vi "AK Befehl Auswerten_v1.2.vi"(10 "Array":string[](array[string])) -> (2 "String für schreiben":string)   [LabVIEW 2020, in "AK-Schnittstelle.lvlib"]
uses:
  AK-Schnittstelle.lvlib
  Aktionen Stoernummern pruefen.ctl
  Aktionen Zustandsfehlerinformation.ctl
  Funktionstasten/Zustaende.ctl
  Funktionstasten/Funktionstasten.lvlib
  Funktionstasten/Betriebsart.ctl
  Funktionstasten/Funktionstasten-Aktion.ctl
  Aktionen Gespeicherte Werte.ctl
  Seiten/Log Konfig/LogKonfig.lvlib
  Seiten/Log Konfig/Aktionen Trigger.ctl
  Seiten/FT-IR/FT-IR.lvlib
  Seiten/FT-IR/FGV FT-IR Gasliste Aktionen.ctl
  Messdaten/Messdaten.lvlib
  Messdaten/Aktionen FGV Messdaten.ctl
  Seiten/System Einstellungen V2/System Einstellungen V2.lvlib
  Seiten/System Einstellungen V2/Aktioen FGV System Konstanten.ctl
  Seiten/Erweiterte Konfig/FGV PID Aktionen.ctl
  Seiten/Erweiterte Konfig/Erweiterte Konfig.lvlib
  Seiten/Erweiterte Konfig/Dichtheitstest.vi
  Allgemein/allgemeine Sub-VIs.lvlib
  cRIO/PC/Kommunikation mit cRIO.lvlib
  Seiten/FT-IR/FGV FT-IR Diagnose Aktionen.ctl
  Seiten/Erweiterte Konfig/Status Dichtheitstest Aktionen.ctl
  Seiten/FT-IR/FGV FT-IR Aktionen.ctl
  Seiten/Anlagengrenzwerte/Anlagengrenzwerte.lvlib
  Seiten/Anlagengrenzwerte/FGV Anlagengrenzwerte Aktionen.ctl
  Seiten/FT-IR/TOOLweb Interface Library/TOOLweb Interface.lvlib
  Seiten/System Einstellungen V2/Aktioen FGV System.ctl
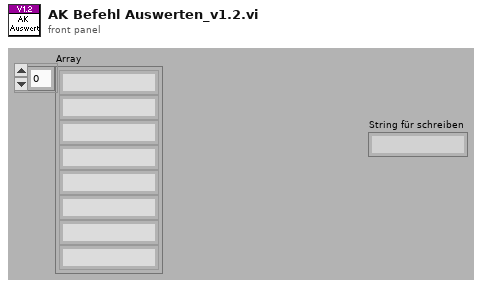
[diagram p1: front panel]
types:
  T1 = typedef "AK-Schnittstelle.lvlib/Aktionen Stoernummern pruefen.ctl" = enum16{"lesen", "prüfen"}
  T2 = typedef "AK-Schnittstelle.lvlib/Aktionen Zustandsfehlerinformation.ctl" = enum16{"OK", "Offline", "Busy", "Syntax Error", "Datenfehler"}
  T3 = typedef "AK-Schnittstelle.lvlib/Aktionen Gespeicherte Werte.ctl" = enum16{"lesen", "laden", "speichern", "Seriell", "TCP", "Diverse", "AKTIV", "AK-Namen"}
  T4 = typedef "System Einstellungen V2.lvlib/Aktioen FGV System Konstanten.ctl" = enum16{"lesen", "laden", "speichern", "Sprache"}
  T5 = typedef "Messdaten.lvlib/Aktionen FGV Messdaten.ctl" = enum16{"lesen", "schreiben", "löschen", "Mittelwerte", "Komponente"}
  T6 = typedef "System Einstellungen V2.lvlib/Aktioen FGV System.ctl" = enum16{"lesen", "laden", "speichern", "Optionen schreiben", "Zeitstempel", "Reset BMP", "Reset SQP", "Wartung", "Werkseinstellung"}
  T7 = typedef "Funktionstasten.lvlib/Funktionstasten-Aktion.ctl" = enum16{"Initialisieren", "Zustand setzen", "Taste gedrückt", "Fehler speichern", "Lesen", "Manuell", "Remote", "Bitparallel", "Samplepoint", "Zeit Prüfen", "reset Umschalten"}
  T8 = typedef "FT-IR.lvlib/FGV FT-IR Gasliste Aktionen.ctl" = enum16{"lesen", "Gasliste FT-IR", "Gasliste ausgelesen", "laden", "speichern", "löschen"}
  T9 = typedef "FT-IR.lvlib/FGV FT-IR Diagnose Aktionen.ctl" = enum16{"Lesen", "Diagnose Schreiben", "Min Schreiben", "Max Schreiben"}
  T10 = typedef "Erweiterte Konfig.lvlib/Status Dichtheitstest Aktionen.ctl" = enum16{"lesen", "Zeitstempel", "Daten", "läuft", "Protokolldaten"}
  T11 = typedef "Erweiterte Konfig.lvlib/FGV PID Aktionen.ctl" = enum16{"Lesen", "Schreiben PID", "Schreiben Sonstige", "Dichtheitstest", "Aktionen Dicht.", "Parameter Sensor"}
  T12 = typedef "FT-IR.lvlib/FGV FT-IR Aktionen.ctl" = enum16{"lesen", "NOG setzen", "NOS setzen", "Initialisieren", "speichern", "ALLES setzen", "FT-IR Spektrum loggen", "Komm Stoppen", "Spektrum LogKonfig"}
  T13 = typedef "Anlagengrenzwerte.lvlib/FGV Anlagengrenzwerte Aktionen.ctl" = enum16{"Lesen", "Grenzwerte schreiben"}
  T14 = typedef "Funktionstasten.lvlib/Zustaende.ctl" = enum16{"Standby", "Pause", "Eco", "Messen", "Kalibrieren", "Spülen Filter", "Spülen Leitung", "Umgebungsluft", "0-Gas", "Cal-Gas", "CG zu PNS", "-------------", "Init 1", "Init 2", "Init 3", "Init 4", "Messen vorbereiten", "Messen durchführen", "Exit"}
  T15 = typedef "Funktionstasten.lvlib/Betriebsart.ctl" = enum16{"Manuell", "Remote", "Bitparallel"}
  T16 = typedef "Funktionstasten.lvlib/Zustaende.ctl" = enum16{"Standby", "Pause", "Eco", "Messen", "Kalibrieren", "Spülen Filter", "Spülen Leitung", "Umgebungsluft", "0-Gas", "Cal-Gas 1", "-------------", "Init 1", "Init 2", "Init 3", "Init 4", "Messen vorbereiten", "Messen durchführen", "Exit"}
  T17 = typedef "LogKonfig.lvlib/Aktionen Trigger.ctl" = enum16{"lesen", "ALLE schreiben", "Trigger prüfen", "Trigger rücksetzen"}
  T18 = typedef "AK-Schnittstelle.lvlib/Diverse gespeicherte Werte.ctl" = cluster{"Kalibriergaseingang":i16, "SamplePoint":i16, "CalGas zu PNS":i16, "Gas-Reihenfolge":i16[], "Zeit 0-Gas":sgl, "Zeit CalGas":sgl, "AK Befehlssatz":T19}
  T19 = typedef "AK-Schnittstelle.lvlib/AK Befehlssatz.ctl" = enum16{"MEXA", "IAG v1.4", "AVL (Puma)", "PEUS"}
  T20 = typedef "System Einstellungen.lvlib/Optionen.ctl" = cluster{"Störmeldep.":bool, "Betriebszustände":bool, "LN2 Befüllung":bool, "Klimaanlage ?":bool, "AK in ppm":bool, "log Cal-Gas":bool, "log 0-Gas":bool, "log CG zu PNS":bool, "Reserve":bool, "Reserve1":bool, "PNS?":bool, "Container":bool, "Mit N2 spülen":bool, "Span Gas Auswahl":T21}
  T21 = typedef "Funktionstasten.lvlib/Spaneingang.ctl" = u16
  T22 = typedef "String - Ausgabefeld.ctl" = string
  T23 = cluster{"AI0: Durchfluss FT-IR":sgl, "AI1: Druck Ausgang":sgl, "AI2: Umgebungsdruck":sgl, "AI3: Druck FT-IR":sgl, "AI4: Druck CalGas":sgl, "AI5: Reserve":sgl, "AI6: Reserve":sgl, "AI7: Reserve":sgl, "Rohwert Durchfluss FT-IR":sgl, "Rohwert Druck Ausgang":sgl, "Rohwert Umgebungsdruck":sgl, "Rohwert Druck FT-IR":sgl, "Rohwert Durchfluss M":sgl, "TC0: Schaltschrank":sgl, "TC1: Filter":sgl, "TC2: Pumpe":sgl, "TC3: HL BMP zu Filter":sgl, "TC4: HL zu FT-IR":sgl, "TC5: HL Extern SP1":sgl, "TC6: HL Extern SP2":sgl, "TC7: Heizung Extern 1":sgl, "TC8: Heizung Extern 2":sgl, "TC9: Reserve":sgl, "TC10: Reserve":sgl, "TC11: Reserve":sgl, "TC12: FT-IR":sgl, "TC13: Reserve":sgl, "TC14: Reserve":sgl, "TC15: Reserve":sgl}
  T24 = typedef "Erweiterte Konfig.lvlib/Sonstige Parameter.ctl" = cluster{"Lüfter langsam":sgl, "Lüfter schnell":sgl, "FT-IR Kühlung Soll":sgl, "FT-IR Kühlung Max":sgl, "Überwachung":T25, "Befüllung aktiv":T26, "Stickstoff Befüllzeit":sgl, "Befüllintervall":sgl, "Kalibrierwert FT-IR":sgl, "Offset Ausgang":sgl, "Offset FT-IR":sgl, "Offset Druck FT-IR":sgl, "Dichtheitstest Zeit":sgl, "Dichtheitstest Abfall":sgl, "Dichtheitstest Umfang":T27, "Offset Umgebung":sgl, "Max Taupunkt":sgl, "Pumpendrehzahl":sgl, "ext. Befüllung":T26, "Ext. Stickstoff Befüllzeit":sgl}
  T25 = typedef "Auswahlfeld.ctl" = u16
  T26 = typedef "LogKonfig.lvlib/Auswahlfeld aktiviert-deaktiviert.ctl" = u16
  T27 = typedef "Erweiterte Konfig.lvlib/Dichtheitstest Umfang.ctl" = u16
  T28 = typedef "Anlagengrenzwerte.lvlib/Anlagen-Grenzwerte Anzeige.ctl" = cluster{"Eingangsdruck FT-IR:":T29, "Durchfluss FT-IR:":T29, "Durchfluss CalGas:":T29, "Druck Ausgang:":T29, "Druck Kalter Block:":T29, "Heizleitungen intern:":T29, "Heizleitung zu FT-IR:":T29, "Heizung Filterblock:":T29, "Heizung Pumpe:":T29, "Heizleitung Extern SP1:":T29, "Heizleitung Extern SP2:":T29, "FT-IR Heizung Messzelle:":T29, "Schaltschranktemperatur:":T29, "Gaskühler:":T29}
  T29 = typedef "Anlagengrenzwerte.lvlib/Anlagen-Parameter Anzeige.ctl" = cluster{"Sollwert":sgl, "Warn-Min":sgl, "Warn-Max":sgl, "Abschalt-Min":sgl, "Abschalt-Max":sgl, "Regler":u16}
  T30 = typedef "LogKonfig.lvlib/Element Triggerereignisse.ctl" = cluster{"Trigger verwenden":T26, "Messwert":u16, "kl./gr.":u16, "Wert":sgl, "Puffergröße":sgl}
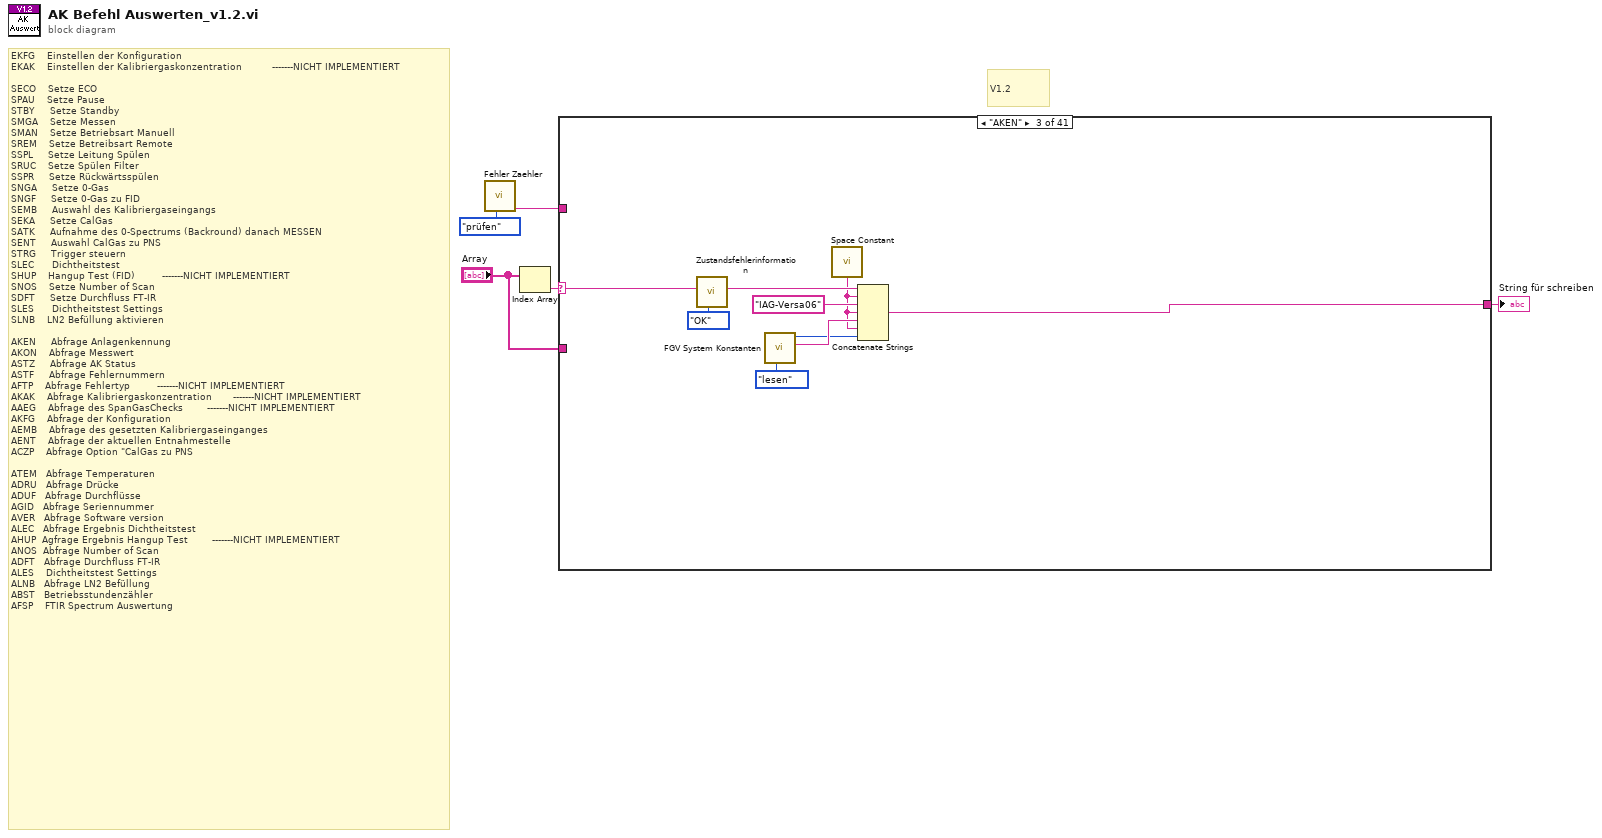
[diagram p0: block diagram]
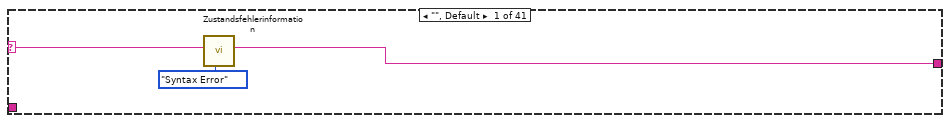
[diagram p2: hidden frame]
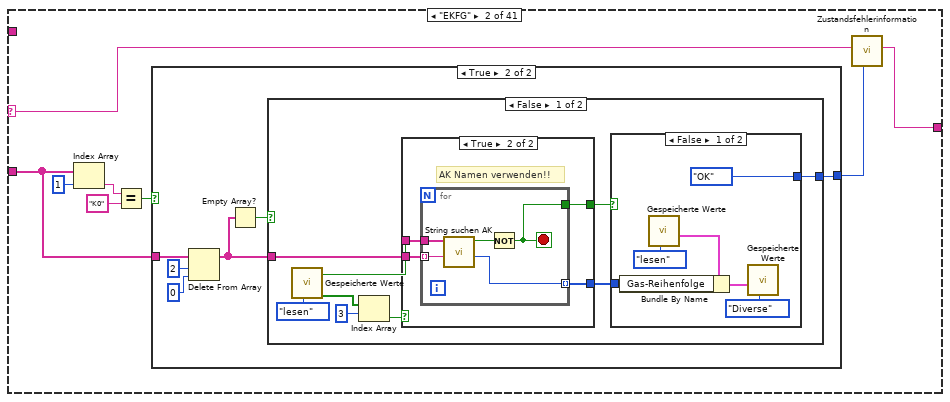
[diagram p3: hidden frame]
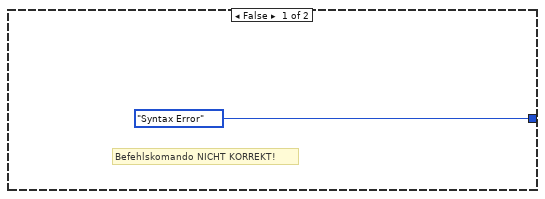
[diagram p4: hidden frame]
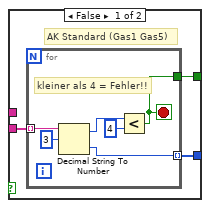
[diagram p5: hidden frame]
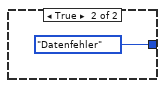
[diagram p6: hidden frame]
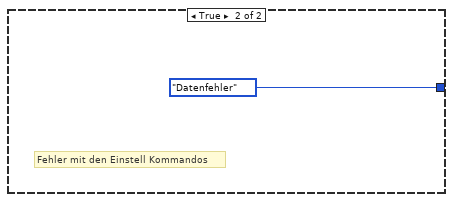
[diagram p7: hidden frame]
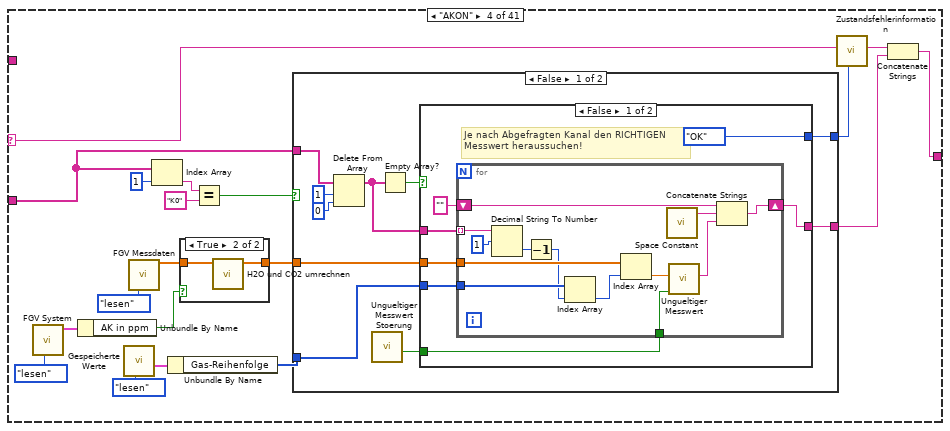
[diagram p8: hidden frame]
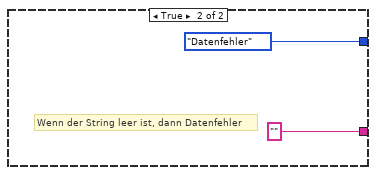
[diagram p10: hidden frame]
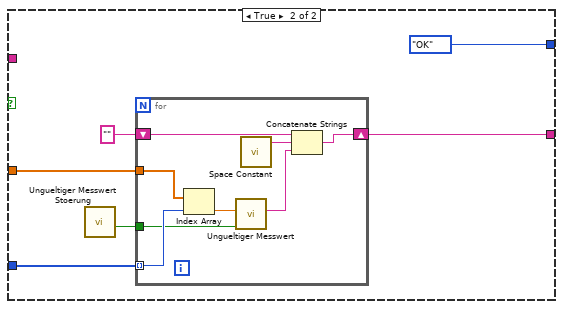
[diagram p11: hidden frame]
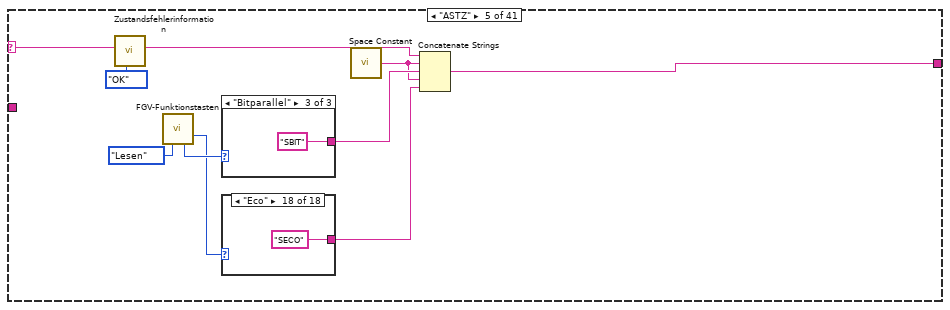
[diagram p12: hidden frame]
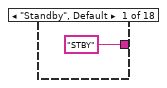
[diagram p13: hidden frame]
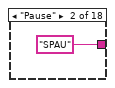
[diagram p14: hidden frame]
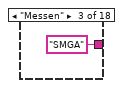
[diagram p15: hidden frame]
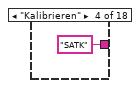
[diagram p16: hidden frame]
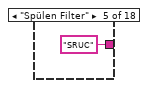
[diagram p17: hidden frame]
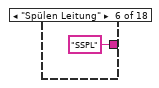
[diagram p18: hidden frame]
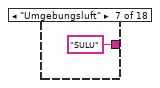
[diagram p19: hidden frame]
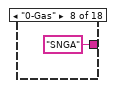
[diagram p20: hidden frame]
diagram:
  # "V1.2"
  # "EKFG    Einstellen der Konfiguration\nEKAK    Einstellen der Kalibriergaskonzentration          -------NICHT IMPLEMENTIERT\n\nSECO    Setze ECO\nSPAU    Setze Pause\nSTBY     Setze Standby\nSMGA    Setze Messen\nSMAN    Setze Betriebsart Manuell\nSREM    Setze Betreibsart Remote\nSSPL     Setze Leitung Spülen\nSRUC    Setze Spülen Filter\nSSPR     Setze Rückwärtsspülen\nSNGA     Setze 0-Gas\nSNGF     Setze 0-Gas zu FID\nSEMB     Auswahl des Kalibriergaseingangs\nSEKA     Setze CalGas\nSATK     Aufnahme des 0-Spectrums (Backround) danach MESSEN\nSENT     Auswahl CalGas zu PNS\nSTRG     Trigger steuern\nSLEC      Dichtheitstest\nSHUP    Hangup Test (FID)         -------NICHT IMPLEMENTIERT\nSNOS    Setze Number of Scan\nSDFT     Setze Durchfluss FT-IR\nSLES      Dichtheitstest Settings\nSLNB    LN2 Befüllung aktivieren\n\nAKEN     Abfrage Anlagenkennung\nAKON    Abfrage Messwert\nASTZ     Abfrage AK Status\nASTF     Abfrage Fehlernummern\nAFTP    Abfrage Fehlertyp         -------NICHT IMPLEMENTIERT\nAKAK    Abfrage Kalibriergaskonzentration       -------NICHT IMPLEMENTIERT\nAAEG    Abfrage des SpanGasChecks        -------NICHT IMPLEMENTIERT\nAKFG    Abfrage der Konfiguration\nAEMB    Abfrage des gesetzten Kalibriergaseinganges\nAENT    Abfrage der aktuellen Entnahmestelle\nACZP    Abfrage Option \"CalGas zu PNS\n\nATEM   Abfrage Temperaturen\nADRU   Abfrage Drücke\nADUF   Abfrage Durchflüsse\nAGID   Abfrage Seriennummer\nAVER   Abfrage Software version\nALEC   Abfrage Ergebnis Dichtheitstest\nAHUP  Agfrage Ergebnis Hangup Test        -------NICHT IMPLEMENTIERT\nANOS  Abfrage Number of Scan\nADFT   Abfrage Durchfluss FT-IR\nALES    Dichtheitstest Settings\nALNB   Abfrage LN2 Befüllung\nABST   Betriebsstundenzähler\nAFSP    FTIR Spectrum Auswertung"
  n1 = call "Fehler Zaehler.vi"("Aktionen"=Aktionen_Stoernummern_pruefen."prüfen") -> ("Fehlerzähler"=w3:string)  [unwired: 7 in, 3 out]
  n2 = Index Array(array="Array") -> (element=w2:string)  [unwired: 1 in]
  n3 = case shown="\"AKEN\"" w2 {
    selector: w2 -> [w7 w15 w65 w85 w143 w163 w176 w223 w232 w241 w257 w280 w294 w301 w308 w323 w344 w355 w364 w374 w388 w396 w399 w402 w405 w415 w425 w429 w439 w443 w445 w458 w463 w484 w503 w507 w529 w568 w592 w643 w674]
    tunnel: [w6 w14 w67 w86 w145 w165 w178 w225 w234 w243 w245 w275 w291 w296 w304 w316 w342 w357 w366 w376 w386 w395 w398 w401 w404 w414 w424 w428 w438 w442 w444 w457 w462 w483 w502 w506 w528 w567 w591 w642 w673] -> w5
    tunnel: w3 -> [_ _ _ _ _ _ _ _ _ _ _ _ _ _ _ _ _ _ _ _ _ _ _ _ _ _ _ _ _ _ _ _ _ _ _ _ _ _ _ _ _]
    tunnel: "Array" -> [_ w16 _ w76 _ _ _ _ _ _ _ _ _ _ _ _ _ _ _ _ _ _ _ _ _ w407 w417 _ w437 _ _ _ w461 _ _ w505 w527 _ w590 w641 w672]
    frame "", Default {
      n4 = call "Zustandsfehlerinformation.vi"("Aktionen"=Aktionen_Zustandsfehlerinformation."Syntax Error", "String"=w7) -> ("String"=w6:string)  [unwired: 9 in]
    }
    frame "EKFG" {
      n5 = Index Array(array=w16, index=1 ("Index")) -> (element=w12:string)
      n6 = Equal?(x=w12, y="K0") -> (x = y?=w10:bool)
      n7 = case shown="True" w10 {
        tunnel: w16 -> [_ w21]
        tunnel: [Aktionen_Zustandsfehlerinformation."Syntax Error" ("Aktionen") w18] -> w9
        frame False {
          # "Befehlskomando NICHT KORREKT!"
        }
        frame True {
          n8 = Delete From Array(array=w21, length=2 ("Länge"), index=0 ("Index")) -> (array with subset deleted=w20:string[])  [unwired: 1 out]
          n9 = Empty Array?(array=w20) -> (empty?=w19:bool)
          n10 = case shown="False" w19 {
            tunnel: w20 -> [w32 _]
            tunnel: [w28 Aktionen_Zustandsfehlerinformation."Datenfehler" ("Aktionen")] -> w18
            frame False {
              n11 = call "Gespeicherte Werte.vi"("Aktionen"=Aktionen_Gespeicherte_Werte."lesen") -> ("AKTIV?"=w25:bool[], "Port changed in"=w29:bool)  [unwired: 5 in, 4 out]
              n12 = Index Array(array=w25, index=3 ("Index")) -> (element=w24:bool)
              n13 = case shown="True" w24 {
                tunnel: w32 -> [w33 w45]
                tunnel: [w34 w44] -> w31
                tunnel: w29 -> [_ w43]
                tunnel: [w35 w42] -> w27
                frame False {
                  # "AK Standard (Gas1 Gas5)"
                  n14 = for {
                    tunnel: w33 -> [w40] mode=indexing
                    tunnel: [w39] -> w34 mode=indexing
                    tunnel: [w36] -> w35
                    stop <- w36 stop-if-true
                    # "kleiner als 4 = Fehler!!"
                    n15 = Decimal String To Number(string=w40, offset=3 ("Offset")) -> (offset past number=w37:i32, number=w39:i32)  [unwired: 1 in]
                    n16 = Less?(x=w37, y=4) -> (x < y?=w36:bool)
                  }
                }
                frame True {
                  # "AK Namen verwenden!!"
                  n17 = for {
                    tunnel: w45 -> [w48] mode=indexing
                    tunnel: [w47] -> w44 mode=indexing
                    tunnel: w43 -> [w49]
                    tunnel: [w50] -> w42
                    stop <- w50 stop-if-true
                    n18 = call "String suchen AK.vi"("gesucht"=w48, "Namen"=w49) -> ("Index"=w47:i32, "Gefunden?"=w46:bool)  [unwired: 8 in]
                    n19 = Not(x=w46) -> (.not. x?=w50:bool)
                  }
                }
              }
              n20 = case shown="False" w27 {
                tunnel: w31 -> [w55 _]
                tunnel: [Aktionen_Zustandsfehlerinformation."OK" ("Aktionen") Aktionen_Zustandsfehlerinformation."Datenfehler" ("Aktionen")] -> w28
                frame False {
                  n21 = call "Gespeicherte Werte.vi"("Aktionen"=Aktionen_Gespeicherte_Werte."lesen") -> ("Diverse Werte"=w53:T18)  [unwired: 6 in, 4 out]
                  n22 = Bundle By Name(cluster=w53, "Gas-Reihenfolge"=w55) -> (w52:T18)
                  n23 = call "Gespeicherte Werte.vi"("Aktionen"=Aktionen_Gespeicherte_Werte."Diverse", "Diverse Werte"=w52) -> ()  [unwired: 5 in, 5 out]
                }
                frame True {
                }
              }
            }
            frame True {
              # "Fehler mit den Einstell Kommandos"
            }
          }
        }
      }
      n24 = call "Zustandsfehlerinformation.vi"("Aktionen"=w9, "String"=w15) -> ("String"=w14:string)  [unwired: 9 in]
    }
    frame "AKEN" {
      n25 = call "Zustandsfehlerinformation.vi"("Aktionen"=Aktionen_Zustandsfehlerinformation."OK", "String"=w65) -> ("String"=w64:string)  [unwired: 9 in]
      n26 = call "FGV System Konstanten.vi"("Aktionen"=Aktioen_FGV_System_Konstanten."lesen") -> ("LanguageList"=w62:string, "Sprachindex"=w61:u16)  [unwired: 6 in, 3 out]
      n27 = call <vilib>:"Space Constant.vi"() -> ("String"=w59:string)
      n28 = Concatenate Strings(w64, w59, "IAG-Versa06" ("String"), w59, w62, w59, w61) -> (w67:string)
    }
    frame "AKON" {
      n29 = call "FGV System.vi"("Aktionen"=Aktioen_FGV_System."lesen") -> ("Optionen"=w70:T20)  [unwired: 8 in, 2 out]
      n30 = Unbundle By Name(w70) -> ("AK in ppm"=w73:bool)
      n31 = call "Gespeicherte Werte.vi"("Aktionen"=Aktionen_Gespeicherte_Werte."lesen") -> ("Diverse Werte"=w74:T18)  [unwired: 6 in, 4 out]
      n32 = call "FGV Messdaten.vi"("Aktionen"=Aktionen_FGV_Messdaten."lesen") -> ("Aktuelle Messwerte"=w72:sgl[])  [unwired: 6 in, 8 out]
      n33 = Index Array(array=w76, index=1 ("Index")) -> (element=w79:string)
      n34 = Unbundle By Name(w74) -> ("Gas-Reihenfolge"=w82:i16[])
      n35 = case shown="True" w73 {
        tunnel: w72 -> [w87 w89]
        tunnel: [w87 w88] -> w69
        frame False {
        }
        frame True {
          n36 = call "H2O und CO2 umrechnen.vi"("Aktuelle Messwerte"=w89) -> ("Aktuelle Messwerte"=w88:sgl[])  [unwired: 10 in]
        }
      }
      n37 = Equal?(x=w79, y="K0") -> (x = y?=w77:bool)
      n38 = case shown="False" w77 {
        tunnel: w82 -> [w93 w127]
        tunnel: [w91 w125] -> w81
        tunnel: w69 -> [w92 w124]
        tunnel: w76 -> [w97 _]
        tunnel: [w95 Aktionen_Zustandsfehlerinformation."OK" ("Aktionen")] -> w75
        frame False {
          n39 = Delete From Array(array=w97, length=1 ("Länge"), index=0 ("Index")) -> (array with subset deleted=w94:string[])  [unwired: 1 out]
          n40 = call "Ungueltiger Messwert Stoerung.vi"() -> ("Störung Messgerät"=w90:bool)  [unwired: 11 in]
          n41 = Empty Array?(array=w94) -> (empty?=w96:bool)
          n42 = case shown="False" w96 {
            tunnel: [Aktionen_Zustandsfehlerinformation."OK" ("Aktionen") Aktionen_Zustandsfehlerinformation."Datenfehler" ("Aktionen")] -> w95
            tunnel: w94 -> [w105 _]
            tunnel: w93 -> [w104 _]
            tunnel: w92 -> [w103 _]
            tunnel: [w102 ""] -> w91
            tunnel: w90 -> [w100 _]
            frame False {
              # "Je nach Abgefragten Kanal den RICHTIGEN\nMesswert heraussuchen!"
              n43 = for {
                tunnel: w105 -> [w119] mode=indexing
                tunnel: w104 -> [w117]
                tunnel: w103 -> [w116]
                shift-right: [w115] -> w102
                shift-left: "" -> [w114]
                tunnel: w100 -> [w108]
                n44 = Decimal String To Number(string=w119, offset=1 ("Offset (0)")) -> (number=w113:i32)  [unwired: 1 in, 1 out]
                n45 = Decrement(x=w113) -> (x-1=w112:i32)
                n46 = Index Array(array=w117, index=w112) -> (element=w110:i16)
                n47 = Index Array(array=w116, index=w110) -> (element=w109:sgl)
                n48 = call <vilib>:"Space Constant.vi"() -> ("String"=w111:string)
                n49 = call "Ungueltiger Messwert.vi"("Stöung Messgerät"=w108, "Messwert"=w109) -> ("Messwert String"=w107:string)  [unwired: 9 in]
                n50 = Concatenate Strings(w114, w111, w107) -> (w115:string)
              }
            }
            frame True {
              # "Wenn der String leer ist, dann Datenfehler"
            }
          }
        }
        frame True {
          n51 = call "Ungueltiger Messwert Stoerung.vi"() -> ("Störung Messgerät"=w122:bool)  [unwired: 11 in]
          n52 = for {
            tunnel: w127 -> [w131] mode=indexing
            shift-right: [w135] -> w125
            shift-left: "" -> [w134]
            tunnel: w124 -> [w133]
            tunnel: w122 -> [w129]
            n53 = Index Array(array=w133, index=w131) -> (element=w130:sgl)
            n54 = call "Ungueltiger Messwert.vi"("Stöung Messgerät"=w129, "Messwert"=w130) -> ("Messwert String"=w128:string)  [unwired: 9 in]
            n55 = call <vilib>:"Space Constant.vi"() -> ("String"=w132:string)
            n56 = Concatenate Strings(w134, w132, w128) -> (w135:string)
          }
        }
      }
      n57 = call "Zustandsfehlerinformation.vi"("Aktionen"=w75, "String"=w85) -> ("String"=w84:string)  [unwired: 9 in]
      n58 = Concatenate Strings(w84, w81) -> (w86:string)
    }
    frame "ASTZ" {
      n59 = call "Zustandsfehlerinformation.vi"("Aktionen"=Aktionen_Zustandsfehlerinformation."OK", "String"=w143) -> ("String"=w142:string)  [unwired: 9 in]
      n60 = call "FGV-Funktionstasten.vi"("Aktion"=Funktionstasten-Aktion."Lesen") -> ("ausgewählte Funktion"=w138:T14, "Betriebsart"=w140:T15)  [unwired: 7 in, 6 out]
      n61 = case shown="\"Bitparallel\"" w140 {
        tunnel: ["SMAN" ("String") "SREM" ("String") "SBIT" ("String")] -> w139
        frame "Manuell", Default {
        }
        frame "Remote" {
        }
        frame "Bitparallel" {
        }
      }
      n62 = case shown="\"Eco\"" w138 {
        tunnel: ["STBY" ("String") "SPAU" ("String") "SMGA" ("String") "SATK" ("String") "SRUC" ("String") "SSPL" ("String") "SULU" ("String") "SNGA" ("String") "SEKA1" ("String") _ _ _ _ _ _ _ _ "SECO" ("String")] -> w136
        frame "Standby", Default {
        }
        frame "Pause" {
        }
        frame "Messen" {
        }
        frame "Kalibrieren" {
        }
        frame "Spülen Filter" {
        }
        frame "Spülen Leitung" {
        }
        frame "Umgebungsluft" {
        }
        frame "0-Gas" {
        }
        frame "Cal-Gas" {
        }
        frame "Init 1" {
        }
        frame "Init 2" {
        }
        frame "-------------" {
        }
        frame "Init 3" {
        }
        frame "Init 4" {
        }
        frame "Messen vorbereiten" {
        }
        frame "Messen durchführen" {
        }
        frame "Exit" {
        }
        frame "Eco" {
        }
      }
      n63 = call <vilib>:"Space Constant.vi"() -> ("String"=w137:string)
      n64 = Concatenate Strings(w142, w137, w139, w137, w136) -> (w145:string)
    }
    frame "ASTF" {
      n65 = call "Zustandsfehlerinformation.vi"("Aktionen"=Aktionen_Zustandsfehlerinformation."OK", "String"=w163) -> ("String"=w162:string)  [unwired: 9 in]
      n66 = call "Fehler Zaehler.vi"("Aktionen"=Aktionen_Stoernummern_pruefen."lesen") -> ("Fehler Nummern"=w160:string)  [unwired: 7 in, 3 out]
      n67 = call <vilib>:"Space Constant.vi"() -> ("String"=w159:string)
      n68 = Concatenate Strings(w162, w159, w160) -> (w165:string)
    }
    frame "AKFG" {
      n69 = call "Gespeicherte Werte.vi"("Aktionen"=Aktionen_Gespeicherte_Werte."lesen") -> ("Diverse Werte"=w172:T18, "Port changed in"=w170:bool)  [unwired: 5 in, 4 out]
      n70 = Unbundle By Name(w172) -> ("Gas-Reihenfolge"=w174:i16[])
      n71 = disable-structure shown="Deaktiviert" {
        disable-tunnel: [w214 _] -> _
        frame Disabled {
          n72 = call "FGV Gasliste.vi"("Aktionen"=FGV_FT-IR_Gasliste_Aktionen."lesen") -> ("Aktuelle Gasliste gesamt"=w214:T22[])  [unwired: 8 in, 2 out]
        }
        frame Enabled {
        }
      }
      n73 = call "Gespeicherte Werte.vi"("Aktionen"=Aktionen_Gespeicherte_Werte."lesen") -> ("AKTIV?"=w169:bool[])  [unwired: 6 in, 4 out]
      n74 = Index Array(array=w169, index=3 ("Index")) -> (element=w166:bool)
      n75 = case shown="True" w166 {
        tunnel: w174 -> [w188 w205]
        tunnel: [w187 w204] -> w171
        tunnel: w170 -> [w186 _]
        frame True {
          n76 = for {
            tunnel: w188 -> [w194] mode=indexing
            shift-right: [w197] -> w187
            shift-left: "" -> [w196]
            tunnel: w186 -> [w195]
            n77 = Index Array(array=w195, index=w194) -> (element=w192)
            n78 = for {
              N: 15 -> [_]
              shift-right: [w202] -> w191
              shift-left: w192 -> [w203]
              stop <- w200 stop-if-true
              n79 = call <vilib>:"Space Constant.vi"() -> ("String"=w199:string)
              n80 = Search and Replace String(input string=w203, search string=w199, replace string="_") -> (result string=w202:string, number of replacements=w201:i32)  [unwired: 5 in, 2 out]
              n81 = Less Or Equal To 0?(x=w201) -> (x <= 0?=w200:bool)
            }
            n82 = call <vilib>:"Space Constant.vi"() -> ("String"=w190:string)
            n83 = Concatenate Strings(w196, w190, w191) -> (w197:string)
          }
        }
        frame False {
          n84 = for {
            tunnel: w205 -> [w210] mode=indexing
            shift-right: [w213] -> w204
            shift-left: "" -> [w212]
            n85 = Number To Decimal String(number=w210) -> (decimal integer string=w208:string)  [unwired: 1 in]
            n86 = Concatenate Strings("Gas" ("String"), w208) -> (w207:string)
            n87 = call <vilib>:"Space Constant.vi"() -> ("String"=w211:string)
            n88 = Concatenate Strings(w212, w211, w207) -> (w213:string)
          }
        }
      }
      n89 = call "Zustandsfehlerinformation.vi"("Aktionen"=Aktionen_Zustandsfehlerinformation."OK", "String"=w176) -> ("String"=w175:string)  [unwired: 9 in]
      n90 = disable-structure shown="Deaktiviert" {
        disable-tunnel: [w185 _] -> _
        disable-tunnel: _ -> [w184 _]
        disable-tunnel: _ -> [w183 _]
        disable-tunnel: _ -> [w181 _]
        frame Disabled {
          n91 = Number To Decimal String(number=w181) -> (decimal integer string=w179:string)  [unwired: 1 in]
          n92 = call <vilib>:"Space Constant.vi"() -> ("String"=w182:string)
          n93 = Concatenate Strings(w184, w182, w183, w182, "K" ("String"), w179) -> (w185:string)
        }
        frame Enabled {
        }
      }
      n94 = Concatenate Strings(w175, w171) -> (w178:string)
    }
    frame "AEMB" {
      n95 = call "Zustandsfehlerinformation.vi"("Aktionen"=Aktionen_Zustandsfehlerinformation."OK", "String"=w223) -> ("String"=w222:string)  [unwired: 9 in]
      n96 = call "Gespeicherte Werte.vi"("Aktionen"=Aktionen_Gespeicherte_Werte."lesen") -> ("Diverse Werte"=w216:T18)  [unwired: 6 in, 4 out]
      n97 = Unbundle By Name(w216) -> ("Kalibriergaseingang"=w220:i16)
      n98 = call <vilib>:"Space Constant.vi"() -> ("String"=w217:string)
      n99 = Number To Decimal String(number=w220) -> (decimal integer string=w218:string)  [unwired: 1 in]
      n100 = Concatenate Strings(w222, w217, "M" ("String"), w218) -> (w225:string)
    }
    frame "AENT" {
      n101 = call "Zustandsfehlerinformation.vi"("Aktionen"=Aktionen_Zustandsfehlerinformation."OK", "String"=w232) -> ("String"=w231:string)  [unwired: 9 in]
      n102 = call "FGV-Funktionstasten.vi"("Aktion"=Funktionstasten-Aktion."Lesen") -> ("Samplepoint"=w226:u16)  [unwired: 7 in, 7 out]
      n103 = call <vilib>:"Space Constant.vi"() -> ("String"=w228:string)
      n104 = Number To Decimal String(number=w226) -> (decimal integer string=w229:string)  [unwired: 1 in]
      n105 = Concatenate Strings(w231, w228, "M" ("String"), w229) -> (w234:string)
    }
    frame "ACZP" {
      n106 = call "Zustandsfehlerinformation.vi"("Aktionen"=Aktionen_Zustandsfehlerinformation."OK", "String"=w241) -> ("String"=w240:string)  [unwired: 9 in]
      n107 = call "Gespeicherte Werte.vi"("Aktionen"=Aktionen_Gespeicherte_Werte."lesen") -> ("Diverse Werte"=w235:T18)  [unwired: 6 in, 4 out]
      n108 = Unbundle By Name(w235) -> ("CalGas zu PNS"=w238:i16)
      n109 = call <vilib>:"Space Constant.vi"() -> ("String"=w236:string)
      n110 = Number To Decimal String(number=w238) -> (decimal integer string=w237:string)  [unwired: 1 in]
      n111 = Concatenate Strings(w240, w236, w237) -> (w243:string)
    }
    frame "ATEM" {
      n112 = call "Zustandsfehlerinformation.vi"("Aktionen"=Aktionen_Zustandsfehlerinformation."OK", "String"=w257) -> ("String"=w244:string)  [unwired: 9 in]
      n113 = call "FGV cRIO-Daten.vi"("Aktion"=enum16{"lesen", "schreiben"}."lesen") -> ("Analog Input"=w255:T23)  [unwired: 6 in, 8 out]
      n114 = Unbundle By Name(w255) -> ("Rohwert Durchfluss M"=w252:sgl, "TC0: Schaltschrank"=w251:sgl, "TC1: Filter"=w250:sgl, "TC2: Pumpe"=w249:sgl, "TC3: HL BMP zu Filter"=w248:sgl, "TC4: HL zu FT-IR"=w247:sgl)
      n115 = call "FGV FT-IR Diagnosewerte.vi"("Aktionen"=FGV_FT-IR_Diagnose_Aktionen."Lesen") -> ("Temperatur"=w253:dbl)  [unwired: 5 in, 5 out]
      n116 = Build Array(w253, w252, w251, w250, w249, w248, w247) -> (w246:dbl[])
      n117 = for {
        tunnel: w246 -> [w264] mode=indexing
        shift-right: [w259] -> w245
        shift-left: w244 -> [w262]
        n118 = Number To Fractional String(number=w264, precision (6)=i16 1 ("Genauigkeit (6)")) -> (F-format string=w260:string)  [unwired: 2 in]
        n119 = call <vilib>:"Space Constant.vi"() -> ("String"=w261:string)
        n120 = Concatenate Strings(w262, w261, w260) -> (w259:string)
      }
    }
    frame "ADRU" {
      n121 = call "Zustandsfehlerinformation.vi"("Aktionen"=Aktionen_Zustandsfehlerinformation."OK", "String"=w280) -> ("String"=w274:string)  [unwired: 9 in]
      n122 = call "FGV cRIO-Daten.vi"("Aktion"=enum16{"lesen", "schreiben"}."lesen") -> ("Analog Input"=w278:T23)  [unwired: 6 in, 8 out]
      n123 = Unbundle By Name(w278) -> ("AI1: Druck Ausgang"=w270:sgl, "AI3: Druck FT-IR"=w268:sgl)
      n124 = call "FGV FT-IR Diagnosewerte.vi"("Aktionen"=FGV_FT-IR_Diagnose_Aktionen."Lesen") -> ("Druck"=w272:dbl)  [unwired: 5 in, 5 out]
      n125 = Number To Fractional String(number=w272, precision (6)=i16 3 ("Genauigkeit (6)")) -> (F-format string=w267:string)  [unwired: 2 in]
      n126 = Number To Fractional String(number=w270, precision (6)=i16 0 ("Genauigkeit (6)")) -> (F-format string=w265:string)  [unwired: 2 in]
      n127 = Number To Fractional String(number=w268, precision (6)=i16 1 ("Genauigkeit (6)")) -> (F-format string=w266:string)  [unwired: 2 in]
      n128 = Build Array(w267, w265, w266) -> (w276:string[])
      n129 = for {
        tunnel: w276 -> [w282] mode=indexing
        shift-right: [w283] -> w275
        shift-left: w274 -> [w285]
        n130 = call <vilib>:"Space Constant.vi"() -> ("String"=w284:string)
        n131 = Concatenate Strings(w285, w284, w282) -> (w283:string)
      }
    }
    frame "ADUF" {
      n132 = call "Zustandsfehlerinformation.vi"("Aktionen"=Aktionen_Zustandsfehlerinformation."OK", "String"=w294) -> ("String"=w290:string)  [unwired: 9 in]
      n133 = call "FGV cRIO-Daten.vi"("Aktion"=enum16{"lesen", "schreiben"}."lesen") -> ("Analog Input"=w293:T23)  [unwired: 6 in, 8 out]
      n134 = Unbundle By Name(w293) -> ("AI0: Durchfluss FT-IR"=w289:sgl)
      n135 = Number To Fractional String(number=w289, precision (6)=i16 1 ("Genauigkeit (6)")) -> (F-format string=w286:string)  [unwired: 2 in]
      n136 = call <vilib>:"Space Constant.vi"() -> ("String"=w287:string)
      n137 = Concatenate Strings(w290, w287, w286) -> (w291:string)
    }
    frame "AGID" {
      n138 = call "Zustandsfehlerinformation.vi"("Aktionen"=Aktionen_Zustandsfehlerinformation."OK", "String"=w301) -> ("String"=w298:string)  [unwired: 9 in]
      n139 = call "FGV System Konstanten.vi"("Aktionen"=Aktioen_FGV_System_Konstanten."lesen") -> ("LanguageList"=w297:string)  [unwired: 6 in, 4 out]
      n140 = call <vilib>:"Space Constant.vi"() -> ("String"=w300:string)
      n141 = Concatenate Strings(w298, w300, w297) -> (w296:string)
    }
    frame "AVER" {
      n142 = call "Zustandsfehlerinformation.vi"("Aktionen"=Aktionen_Zustandsfehlerinformation."OK", "String"=w308) -> ("String"=w305:string)  [unwired: 9 in]
      n143 = call "FGV System Konstanten.vi"("Aktionen"=Aktioen_FGV_System_Konstanten."lesen") -> ("Sprachindex"=w303:u16)  [unwired: 6 in, 4 out]
      n144 = call <vilib>:"Space Constant.vi"() -> ("String"=w307:string)
      n145 = Concatenate Strings(w305, w307, w303) -> (w304:string)
    }
    frame "ALEC" {
      n146 = call "Zustandsfehlerinformation.vi"("Aktionen"=Aktionen_Zustandsfehlerinformation."OK", "String"=w323) -> ("String"=w322:string)  [unwired: 9 in]
      n147 = call "Status Dichtheitstest.vi"("Aktionen"=Status_Dichtheitstest_Aktionen."lesen") -> ("Fehler"=w311:bool, "läuft?"=w315:bool, "Anstieg"=w320:sgl)  [unwired: 6 in, 2 out]
      n148 = Or(x=w315, y=w311) -> (x .or. y?=w314:bool)
      n149 = Number To Decimal String(number=w320) -> (decimal integer string=w319:string)  [unwired: 1 in]
      n150 = call <vilib>:"Space Constant.vi"() -> ("String"=w318:string)
      n151 = Concatenate Strings(w322, w318, w319) -> (w317:string)
      n152 = Select(t="error", s=w311, f="busy") -> (s? t:f=w310:string)
      n153 = case shown="True" w314 {
        tunnel: w317 -> [w325 w328]
        tunnel: [w325 w326] -> w316
        tunnel: w310 -> [_ w327]
        frame False {
        }
        frame True {
          n154 = call <vilib>:"Space Constant.vi"() -> ("String"=w329:string)
          n155 = Concatenate Strings(w328, w329, w327) -> (w326:string)
        }
      }
    }
    frame "ALES" {
      n156 = call "FGV Erweiterte Konfig.vi"("Aktion"=FGV_PID_Aktionen."Lesen") -> ("Sonstige"=w336:T24)  [unwired: 5 in, 5 out]
      n157 = call "Zustandsfehlerinformation.vi"("Aktionen"=Aktionen_Zustandsfehlerinformation."OK", "String"=w344) -> ("String"=w341:string)  [unwired: 9 in]
      n158 = Unbundle By Name(w336) -> ("Dichtheitstest Zeit"=w333:sgl, "Dichtheitstest Abfall"=w332:sgl, "Dichtheitstest Umfang"=w331:T27)
      n159 = Number To Fractional String(number=w333, precision (6)=i16 0 ("Genauigkeit (6)")) -> (F-format string=w330:string)  [unwired: 2 in]
      n160 = Number To Fractional String(number=w332, precision (6)=i16 0 ("Genauigkeit (6)")) -> (F-format string=w337:string)  [unwired: 2 in]
      n161 = Number To Fractional String(number=w331, precision (6)=i16 0 ("Genauigkeit (6)")) -> (F-format string=w338:string)  [unwired: 2 in]
      n162 = Build Array(w330, w337, w338) -> (w343:string[])
      n163 = for {
        tunnel: w343 -> [w346] mode=indexing
        shift-right: [w347] -> w342
        shift-left: w341 -> [w349]
        n164 = call <vilib>:"Space Constant.vi"() -> ("String"=w348:string)
        n165 = Concatenate Strings(w349, w348, w346) -> (w347:string)
      }
    }
    frame "ANOS" {
      n166 = call "Zustandsfehlerinformation.vi"("Aktionen"=Aktionen_Zustandsfehlerinformation."OK", "String"=w355) -> ("String"=w354:string)  [unwired: 9 in]
      n167 = call "FGV FT-IR Parameter.vi"("Aktion"=FGV_FT-IR_Aktionen."lesen") -> ("NoOfScan"=w350:u32)  [unwired: 11 in, 7 out]
      n168 = call <vilib>:"Space Constant.vi"() -> ("String"=w353:string)
      n169 = Number To Decimal String(number=w350) -> (decimal integer string=w352:string)  [unwired: 1 in]
      n170 = Concatenate Strings(w354, w353, w352) -> (w357:string)
    }
    frame "ALNB" {
      n171 = call "Zustandsfehlerinformation.vi"("Aktionen"=Aktionen_Zustandsfehlerinformation."OK", "String"=w364) -> ("String"=w363:string)  [unwired: 9 in]
      n172 = call "FGV Erweiterte Konfig.vi"("Aktion"=FGV_PID_Aktionen."Lesen") -> ("Sonstige"=w360:T24)  [unwired: 5 in, 5 out]
      n173 = Unbundle By Name(w360) -> ("Befüllung aktiv"=w358:T26)
      n174 = call <vilib>:"Space Constant.vi"() -> ("String"=w362:string)
      n175 = Number To Decimal String(number=w358) -> (decimal integer string=w361:string)  [unwired: 1 in]
      n176 = Concatenate Strings(w363, w362, w361) -> (w366:string)
    }
    frame "ADFT" {
      n177 = call "FGV Anlagengrenzwerte.vi"("Aktion"=FGV_Anlagengrenzwerte_Aktionen."Lesen") -> ("Anlagen-Grenzwerte Anzeige"=w370:T28)  [unwired: 1 in, 9 out]
      n178 = call "Zustandsfehlerinformation.vi"("Aktionen"=Aktionen_Zustandsfehlerinformation."OK", "String"=w374) -> ("String"=w373:string)  [unwired: 9 in]
      n179 = Unbundle By Name(w370) -> ("Durchfluss FT-IR:.Sollwert"=w369:sgl)
      n180 = call <vilib>:"Space Constant.vi"() -> ("String"=w372:string)
      n181 = Number To Fractional String(number=w369, precision (6)=i16 1 ("Genauigkeit (6)")) -> (F-format string=w367:string)  [unwired: 2 in]
      n182 = Concatenate Strings(w373, w372, w367) -> (w376:string)
    }
    frame "ABST" {
      n183 = call "Zustandsfehlerinformation.vi"("Aktionen"=Aktionen_Zustandsfehlerinformation."OK", "String"=w388) -> ("String"=w385:string)  [unwired: 9 in]
      n184 = call "FGV cRIO-Daten.vi"("Aktion"=enum16{"lesen", "schreiben"}."lesen") -> ("PID Stellwerte"=w377:i16[])  [unwired: 6 in, 8 out]
      n185 = Index Array(array=w377) -> (element #1=w378:i16, element #2=w379:i16)  [unwired: 2 in]
      n186 = Number To Fractional String(number=w378, precision (6)=i16 1 ("Genauigkeit (6)")) -> (F-format string=w382:string)  [unwired: 2 in]
      n187 = Number To Fractional String(number=w379, precision (6)=i16 1 ("Genauigkeit (6)")) -> (F-format string=w381:string)  [unwired: 2 in]
      n188 = Build Array(w382, w381) -> (w387:string[])
      n189 = for {
        tunnel: w387 -> [w390] mode=indexing
        shift-right: [w391] -> w386
        shift-left: w385 -> [w393]
        n190 = call <vilib>:"Space Constant.vi"() -> ("String"=w392:string)
        n191 = Concatenate Strings(w393, w392, w390) -> (w391:string)
      }
    }
    frame "SECO" {
      n192 = call "Setze Zustand.vi"("AK Befehl"=w396, "Zustand"=Zustaende."Pause") -> ("Antwort String"=w395:string)  [unwired: 8 in, 1 out]
    }
    frame "SPAU" {
      n193 = call "Setze Zustand.vi"("AK Befehl"=w399, "Zustand"=Zustaende."Pause") -> ("Antwort String"=w398:string)  [unwired: 8 in, 1 out]
    }
    frame "STBY" {
      n194 = call "Setze Zustand.vi"("AK Befehl"=w402, "Zustand"=Zustaende."Standby") -> ("Antwort String"=w401:string)  [unwired: 8 in, 1 out]
    }
    frame "SMGA" {
      n195 = call "Setze Zustand.vi"("AK Befehl"=w405, "Zustand"=Zustaende."Messen") -> ("Antwort String"=w404:string)  [unwired: 8 in, 1 out]
    }
    frame "SSPL" {
      n196 = Index Array(array=w407, index=2 ("Index")) -> (element=w411:string)
      n197 = Decimal String To Number(string=w411) -> (number=w410:i32)  [unwired: 2 in, 1 out]
      n198 = Divide(x=w410, y=10) -> (x/y=w408:dbl)
      n199 = To Single Precision Float(number=w408) -> (single precision float=w406:sgl)
      n200 = call "Setze Zustand.vi"("Zeit"=w406, "AK Befehl"=w415, "Zustand"=Zustaende."Spülen Leitung") -> ("Antwort String"=w414:string)  [unwired: 7 in, 1 out]
    }
    frame "SRUC" {
      n201 = Index Array(array=w417, index=2 ("Index")) -> (element=w421:string)
      n202 = Decimal String To Number(string=w421) -> (number=w420:i32)  [unwired: 2 in, 1 out]
      n203 = Divide(x=w420, y=10) -> (x/y=w418:dbl)
      n204 = To Single Precision Float(number=w418) -> (single precision float=w416:sgl)
      n205 = call "Setze Zustand.vi"("Zeit"=w416, "AK Befehl"=w425, "Zustand"=Zustaende."Spülen Filter") -> ("Antwort String"=w424:string)  [unwired: 7 in, 1 out]
    }
    frame "SSPR" {
      n206 = call "Setze Zustand.vi"("Befehl nicht vorhanden!"=TRUE, "AK Befehl"=w429, "Zustand"=Zustaende."Standby") -> ("Antwort String"=w428:string)  [unwired: 7 in, 1 out]
    }
    frame "SNGA" {
      n207 = Index Array(array=w437, index=2 ("Index")) -> (element=w435:string)
      n208 = Decimal String To Number(string=w435) -> (number=w434:i32)  [unwired: 2 in, 1 out]
      n209 = Divide(x=w434, y=10) -> (x/y=w432:dbl)
      n210 = To Single Precision Float(number=w432) -> (single precision float=w430:sgl)
      n211 = call "Setze Zustand.vi"("Zeit"=w430, "AK Befehl"=w439, "Zustand"=Zustaende."0-Gas") -> ("Antwort String"=w438:string)  [unwired: 7 in, 1 out]
    }
    frame "SNGF" {
      n212 = call "Setze Zustand.vi"("Befehl nicht vorhanden!"=TRUE, "AK Befehl"=w443, "Zustand"=Zustaende."Standby") -> ("Antwort String"=w442:string)  [unwired: 7 in, 1 out]
    }
    frame "SMAN" {
      n213 = call "FGV-Funktionstasten.vi"("Aktion"=Funktionstasten-Aktion."Lesen") -> ("Betriebsart"=w449:T15)  [unwired: 7 in, 7 out]
      n214 = Equal?(x=w449, y=Betriebsart."Remote" ("Betriebsart")) -> (x = y?=w446:bool)
      n215 = case shown="True" w446 {
        tunnel: w445 -> [w452 w455]
        tunnel: [w450 w454] -> w444
        frame False {
          n216 = call "Zustandsfehlerinformation.vi"("Aktionen"=Aktionen_Zustandsfehlerinformation."Offline", "String"=w452) -> ("String"=w450:string)  [unwired: 9 in]
        }
        frame True {
          n217 = call "Zustandsfehlerinformation.vi"("Aktionen"=Aktionen_Zustandsfehlerinformation."OK", "String"=w455) -> ("String"=w454:string)  [unwired: 9 in]
          n218 = call "FGV-Funktionstasten.vi"("Aktion"=Funktionstasten-Aktion."Manuell") -> ()  [unwired: 7 in, 8 out]
        }
      }
    }
    frame "SREM" {
      n219 = call "Zustandsfehlerinformation.vi"("Aktionen"=Aktionen_Zustandsfehlerinformation."OK", "String"=w458) -> ("String"=w457:string)  [unwired: 9 in]
      n220 = call "FGV-Funktionstasten.vi"("Aktion"=Funktionstasten-Aktion."Remote") -> ()  [unwired: 7 in, 8 out]
    }
    frame "SEMB" {
      n221 = call "FGV-Funktionstasten.vi"("Aktion"=Funktionstasten-Aktion."Lesen") -> ("Betriebsart"=w466:T15)  [unwired: 7 in, 7 out]
      n222 = Equal?(x=w466, y=Betriebsart."Remote" ("Betriebsart")) -> (x = y?=w467:bool)
      n223 = case shown="True" w467 {
        tunnel: w463 -> [w469 w481]
        tunnel: [w468 w480] -> w462
        tunnel: w461 -> [_ w479]
        frame False {
          n224 = call "Zustandsfehlerinformation.vi"("Aktionen"=Aktionen_Zustandsfehlerinformation."Offline", "String"=w469) -> ("String"=w468:string)  [unwired: 9 in]
        }
        frame True {
          n225 = Index Array(array=w479, index=2 ("Index")) -> (element=w477:string)
          n226 = call "Zustandsfehlerinformation.vi"("Aktionen"=Aktionen_Zustandsfehlerinformation."OK", "String"=w481) -> ("String"=w480:string)  [unwired: 9 in]
          n227 = Decimal String To Number(string=w477, offset=1 ("Offset (0)")) -> (number=w473:i32)  [unwired: 1 in, 1 out]
          n228 = call "Gespeicherte Werte.vi"("Aktionen"=Aktionen_Gespeicherte_Werte."lesen") -> ("Diverse Werte"=w472:T18)  [unwired: 6 in, 4 out]
          n229 = Bundle By Name(cluster=w472, "Kalibriergaseingang"=w473) -> (w471:T18)
          n230 = call "Gespeicherte Werte.vi"("Aktionen"=Aktionen_Gespeicherte_Werte."Diverse", "Diverse Werte"=w471) -> ()  [unwired: 5 in, 5 out]
        }
      }
    }
    frame "SEKA" {
      n231 = call "FGV-Funktionstasten.vi"("Aktion"=Funktionstasten-Aktion."Lesen") -> ("Betriebsart"=w487:T15)  [unwired: 7 in, 7 out]
      n232 = Equal?(x=w487, y=Betriebsart."Remote" ("Betriebsart")) -> (x = y?=w488:bool)
      n233 = case shown="True" w488 {
        tunnel: w484 -> [w490 w494]
        tunnel: [w489 w493] -> w483
        frame False {
          n234 = call "Zustandsfehlerinformation.vi"("Aktionen"=Aktionen_Zustandsfehlerinformation."Offline", "String"=w490) -> ("String"=w489:string)  [unwired: 9 in]
        }
        frame True {
          n235 = call "Gespeicherte Werte.vi"("Aktionen"=Aktionen_Gespeicherte_Werte."lesen") -> ("Diverse Werte"=w496:T18)  [unwired: 6 in, 4 out]
          n236 = Unbundle By Name(w496) -> ("Kalibriergaseingang"=w495:i16)
          n237 = case shown="3" w495 {
            tunnel: [Zustaende."Standby" ("Zustand") Zustaende."Cal-Gas 1" ("Zustand") Zustaende."-------------" ("Zustand") Zustaende."Init 1" ("Zustand")] -> w492
            frame 0, Default {
            }
            frame 1 {
            }
            frame 2 {
            }
            frame 3 {
            }
          }
          n238 = call "Setze Zustand.vi"("AK Befehl"=w494, "Zustand"=w492) -> ("Antwort String"=w493:string)  [unwired: 8 in, 1 out]
        }
      }
    }
    frame "SATK" {
      n239 = call "Setze Zustand.vi"("AK Befehl"=w503, "Zustand"=Zustaende."Kalibrieren") -> ("Antwort String"=w502:string)  [unwired: 8 in, 1 out]
    }
    frame "SENT" {
      n240 = call "FGV-Funktionstasten.vi"("Aktion"=Funktionstasten-Aktion."Lesen") -> ("Betriebsart"=w510:T15)  [unwired: 7 in, 7 out]
      n241 = Equal?(x=w510, y=Betriebsart."Remote" ("Betriebsart")) -> (x = y?=w511:bool)
      n242 = case shown="True" w511 {
        tunnel: w507 -> [w513 w525]
        tunnel: [w512 w524] -> w506
        tunnel: w505 -> [_ w523]
        frame False {
          n243 = call "Zustandsfehlerinformation.vi"("Aktionen"=Aktionen_Zustandsfehlerinformation."Offline", "String"=w513) -> ("String"=w512:string)  [unwired: 9 in]
        }
        frame True {
          n244 = Index Array(array=w523, index=2 ("Index")) -> (element=w521:string)
          n245 = call "Zustandsfehlerinformation.vi"("Aktionen"=Aktionen_Zustandsfehlerinformation."OK", "String"=w525) -> ("String"=w524:string)  [unwired: 9 in]
          n246 = Decimal String To Number(string=w521) -> (number=w515:i32)  [unwired: 2 in, 1 out]
          n247 = call "FGV-Funktionstasten.vi"("Samplepoint"=w515, "Aktion"=Funktionstasten-Aktion."Samplepoint") -> ()  [unwired: 6 in, 8 out]
          n248 = call "Gespeicherte Werte.vi"("Aktionen"=Aktionen_Gespeicherte_Werte."lesen") -> ("Diverse Werte"=w518:T18)  [unwired: 6 in, 4 out]
          n249 = Bundle By Name(cluster=w518, "SamplePoint"=w515) -> (w517:T18)
          n250 = call "Gespeicherte Werte.vi"("Aktionen"=Aktionen_Gespeicherte_Werte."Diverse", "Diverse Werte"=w517) -> ()  [unwired: 5 in, 5 out]
        }
      }
    }
    frame "STRG" {
      n251 = call "FGV-Funktionstasten.vi"("Aktion"=Funktionstasten-Aktion."Lesen") -> ("Betriebsart"=w532:T15)  [unwired: 7 in, 7 out]
      n252 = Equal?(x=w532, y=Betriebsart."Remote" ("Betriebsart")) -> (x = y?=w533:bool)
      n253 = case shown="False" w533 {
        tunnel: w529 -> [w535 w542]
        tunnel: [w534 w541] -> w528
        tunnel: w527 -> [_ w540]
        frame False {
          n254 = call "Zustandsfehlerinformation.vi"("Aktionen"=Aktionen_Zustandsfehlerinformation."Offline", "String"=w535) -> ("String"=w534:string)  [unwired: 9 in]
        }
        frame True {
          n255 = Index Array(array=w540, index=2 ("Index")) -> (element=w538:string)
          n256 = Empty String/Path?(string/path=w538) -> (empty?=w537:bool)
          n257 = case shown="False" w537 {
            tunnel: w542 -> [w549 w562]
            tunnel: [w548 w561] -> w541
            tunnel: w538 -> [w547 _]
            frame False {
              n258 = Decimal String To Number(string=w547) -> (number=w544:i32)  [unwired: 2 in, 1 out]
              n259 = In Range and Coerce(upper limit=2 ("Obergrenze"), x=w544, lower limit=0 ("Untergrenze")) -> (In Range?=w543:bool)  [unwired: 1 out]
              n260 = case shown="True" w543 {
                tunnel: w549 -> [w551 w559]
                tunnel: [w550 w558] -> w548
                tunnel: w544 -> [_ w553]
                frame False {
                  n261 = call "Zustandsfehlerinformation.vi"("Aktionen"=Aktionen_Zustandsfehlerinformation."Datenfehler", "String"=w551) -> ("String"=w550:string)  [unwired: 9 in]
                }
                frame True {
                  # "Wenn informationen da sind, dann übergeben!"
                  n262 = call "FGV Trigger.vi"("Aktion"=Aktionen_Trigger."lesen") -> ("Triggerereignis neu"=w555:T30)  [unwired: 7 in, 3 out]
                  n263 = Bundle By Name(cluster=w555, "Trigger verwenden"=w553) -> (w554:T30)
                  n264 = call "Zustandsfehlerinformation.vi"("Aktionen"=Aktionen_Zustandsfehlerinformation."OK", "String"=w559) -> ("String"=w558:string)  [unwired: 9 in]
                  n265 = call "FGV Trigger.vi"("Aktion"=Aktionen_Trigger."ALLE schreiben", "Triggerereignis"=w554) -> ()  [unwired: 6 in, 4 out]
                }
              }
            }
            frame True {
              # "Wenn nur STRG dann Trigger setzen!!!"
              n266 = call "FGV Trigger.vi"("Aktion"=Aktionen_Trigger."Trigger prüfen", "Trigger setzen"=TRUE) -> ()  [unwired: 6 in, 4 out]
              n267 = call "Zustandsfehlerinformation.vi"("Aktionen"=Aktionen_Zustandsfehlerinformation."OK", "String"=w562) -> ("String"=w561:string)  [unwired: 9 in]
            }
          }
        }
      }
    }
    frame "SLEC" {
      n268 = call "FGV-Funktionstasten.vi"("Aktion"=Funktionstasten-Aktion."Lesen") -> ("ausgewählte Funktion"=w566:T14, "Betriebsart"=w571:T15)  [unwired: 7 in, 6 out]
      n269 = Equal?(x=w571, y=Betriebsart."Remote" ("Betriebsart")) -> (x = y?=w572:bool)
      n270 = case shown="True" w572 {
        tunnel: w568 -> [w574 w580]
        tunnel: [w573 w579] -> w567
        tunnel: w566 -> [_ w578]
        frame False {
          n271 = call "Zustandsfehlerinformation.vi"("Aktionen"=Aktionen_Zustandsfehlerinformation."Offline", "String"=w574) -> ("String"=w573:string)  [unwired: 9 in]
        }
        frame True {
          n272 = Equal?(x=w578, y=Zustaende."Standby") -> (x = y?=w576:bool)
          n273 = case shown="True" w576 {
            tunnel: w580 -> [w583 w585]
            tunnel: [w582 w584] -> w579
            frame False {
              n274 = call "Zustandsfehlerinformation.vi"("Aktionen"=Aktionen_Zustandsfehlerinformation."Datenfehler", "String"=w583) -> ("String"=w582:string)  [unwired: 9 in]
            }
            frame True {
              n275 = flat-sequence {
                frame #0 {
                  n276 = call "FGV Erweiterte Konfig.vi"("Aktion"=FGV_PID_Aktionen."Dichtheitstest", "Dichtheitstest?"=TRUE) -> ()  [unwired: 5 in, 5 out]
                }
                frame #1 {
                  n277 = vi-ref "Erweiterte Konfig.lvlib:Dichtheitstest.vi"() -> (w589:refnum<vi>)
                  n278 = call "VI Pop Up.vi"("VI Referenz"=w589) -> ()  [unwired: 11 in]
                }
              }
              n279 = call "Zustandsfehlerinformation.vi"("Aktionen"=Aktionen_Zustandsfehlerinformation."OK", "String"=w585) -> ("String"=w584:string)  [unwired: 9 in]
            }
          }
        }
      }
    }
    frame "SLES" {
      n280 = call "FGV-Funktionstasten.vi"("Aktion"=Funktionstasten-Aktion."Lesen") -> ("Betriebsart"=w595:T15)  [unwired: 7 in, 7 out]
      n281 = Equal?(x=w595, y=Betriebsart."Remote" ("Betriebsart")) -> (x = y?=w596:bool)
      n282 = case shown="True" w596 {
        tunnel: w592 -> [w598 w631]
        tunnel: [w597 w630] -> w591
        tunnel: w590 -> [_ w629]
        frame False {
          n283 = call "Zustandsfehlerinformation.vi"("Aktionen"=Aktionen_Zustandsfehlerinformation."Offline", "String"=w598) -> ("String"=w597:string)  [unwired: 9 in]
        }
        frame True {
          n284 = Index Array(array=w629, index #1=2 ("Index"), index #2=3 ("Index"), index #3=4 ("Index")) -> (element #1=w603:string, element #2=w604:string, element #3=w605:string)
          n285 = Empty String/Path?(string/path=w603) -> (empty?=w608:bool)
          n286 = Empty String/Path?(string/path=w604) -> (empty?=w607:bool)
          n287 = Empty String/Path?(string/path=w605) -> (empty?=w606:bool)
          n288 = Decimal String To Number(string=w603) -> (number=w625:i32)  [unwired: 2 in, 1 out]
          n289 = Decimal String To Number(string=w604) -> (number=w621:i32)  [unwired: 2 in, 1 out]
          n290 = Decimal String To Number(string=w605) -> (number=w616:i32)  [unwired: 2 in, 1 out]
          n291 = Not(x=w608) -> (.not. x?=w602:bool)
          n292 = Not(x=w607) -> (.not. x?=w601:bool)
          n293 = Not(x=w606) -> (.not. x?=w600:bool)
          n294 = In Range and Coerce(upper limit=101 ("Obergrenze"), x=w625, lower limit=1 ("Untergrenze")) -> (coerced(x)=w611:i32, In Range?=w613:bool)
          n295 = In Range and Coerce(upper limit=101 ("Obergrenze"), x=w621, lower limit=1 ("Untergrenze")) -> (coerced(x)=w610:i32, In Range?=w614:bool)
          n296 = In Range and Coerce(upper limit=3 ("Obergrenze"), x=w616, lower limit=0 ("Untergrenze")) -> (coerced(x)=w609:i32, In Range?=w615:bool)
          n297 = Compound Arithmetic op=AND(w613, w614, w615, w602, w601, w600) -> (w612:bool)
          n298 = case shown="True" w612 {
            tunnel: [Aktionen_Zustandsfehlerinformation."Datenfehler" ("Aktionen") Aktionen_Zustandsfehlerinformation."OK" ("Aktionen")] -> w624
            tunnel: w611 -> [_ w635]
            tunnel: w610 -> [_ w634]
            tunnel: w609 -> [_ w633]
            frame False {
            }
            frame True {
              n299 = call "FGV Erweiterte Konfig.vi"("Aktion"=FGV_PID_Aktionen."Lesen") -> ("Sonstige"=w638:T24)  [unwired: 5 in, 5 out]
              n300 = Bundle By Name(cluster=w638, "Dichtheitstest Zeit"=w635, "Dichtheitstest Abfall"=w634, "Dichtheitstest Umfang"=w633) -> (w639:T24)
              n301 = call "FGV Erweiterte Konfig.vi"("Aktion"=FGV_PID_Aktionen."Schreiben Sonstige", "Sonstige"=w639) -> ()  [unwired: 4 in, 6 out]
            }
          }
          n302 = call "Zustandsfehlerinformation.vi"("Aktionen"=w624, "String"=w631) -> ("String"=w630:string)  [unwired: 9 in]
        }
      }
    }
    frame "SLNB" {
      n303 = call "FGV-Funktionstasten.vi"("Aktion"=Funktionstasten-Aktion."Lesen") -> ("Betriebsart"=w646:T15)  [unwired: 7 in, 7 out]
      n304 = Equal?(x=w646, y=Betriebsart."Remote" ("Betriebsart")) -> (x = y?=w647:bool)
      n305 = case shown="True" w647 {
        tunnel: w643 -> [w649 w664]
        tunnel: [w648 w663] -> w642
        tunnel: w641 -> [_ w662]
        frame False {
          n306 = call "Zustandsfehlerinformation.vi"("Aktionen"=Aktionen_Zustandsfehlerinformation."Offline", "String"=w649) -> ("String"=w648:string)  [unwired: 9 in]
        }
        frame True {
          # "0 oder 1"
          n307 = Index Array(array=w662, index=2 ("Index")) -> (element=w653:string)
          n308 = Decimal String To Number(string=w653) -> (number=w658:i32)  [unwired: 2 in, 1 out]
          n309 = Empty String/Path?(string/path=w653) -> (empty?=w652:bool)
          n310 = In Range and Coerce(upper limit=2 ("Obergrenze"), x=w658, lower limit=0 ("Untergrenze")) -> (coerced(x)=w654:i32, In Range?=w656:bool)
          n311 = Not(x=w652) -> (.not. x?=w651:bool)
          n312 = And(x=w656, y=w651) -> (x .and. y?=w655:bool)
          n313 = case shown="True" w655 {
            tunnel: [Aktionen_Zustandsfehlerinformation."Datenfehler" ("Aktionen") Aktionen_Zustandsfehlerinformation."OK" ("Aktionen")] -> w657
            tunnel: w654 -> [_ w666]
            frame False {
            }
            frame True {
              n314 = call "FGV Erweiterte Konfig.vi"("Aktion"=FGV_PID_Aktionen."Lesen") -> ("Sonstige"=w669:T24)  [unwired: 5 in, 5 out]
              n315 = Bundle By Name(cluster=w669, "Befüllung aktiv"=w666) -> (w670:T24)
              n316 = call "FGV Erweiterte Konfig.vi"("Aktion"=FGV_PID_Aktionen."Schreiben Sonstige", "Sonstige"=w670) -> ()  [unwired: 4 in, 6 out]
            }
          }
          n317 = call "Zustandsfehlerinformation.vi"("Aktionen"=w657, "String"=w664) -> ("String"=w663:string)  [unwired: 9 in]
        }
      }
    }
    frame "SNOS" {
      n318 = call "FGV-Funktionstasten.vi"("Aktion"=Funktionstasten-Aktion."Lesen") -> ("Betriebsart"=w677:T15)  [unwired: 7 in, 7 out]
      n319 = Equal?(x=w677, y=Betriebsart."Remote" ("Betriebsart")) -> (x = y?=w678:bool)
      n320 = case shown="True" w678 {
        tunnel: w674 -> [w680 w692]
        tunnel: [w679 w691] -> w673
        tunnel: w672 -> [_ w690]
        frame False {
          n321 = call "Zustandsfehlerinformation.vi"("Aktionen"=Aktionen_Zustandsfehlerinformation."Offline", "String"=w680) -> ("String"=w679:string)  [unwired: 9 in]
        }
        frame True {
          n322 = Index Array(array=w690, index=2 ("Index")) -> (element=w688:string)
          n323 = Decimal String To Number(string=w688) -> (number=w685:i32)  [unwired: 2 in, 1 out]
          n324 = In Range and Coerce(upper limit=101 ("Obergrenze"), x=w685, lower limit=1 ("Untergrenze")) -> (coerced(x)=w684:i32, In Range?=w683:bool)
          n325 = case shown="True" w683 {
            tunnel: w684 -> [_ w694]
            tunnel: [Aktionen_Zustandsfehlerinformation."Datenfehler" ("Aktionen") Aktionen_Zustandsfehlerinformation."OK" ("Aktionen")] -> w682
            frame False {
            }
            frame True {
              n326 = flat-sequence {
                tunnel: w694 -> [w696]
                frame #0 {
                  n327 = call "FGV FT-IR Parameter.vi"("NoOfScan neu"=w696, "Aktion"=FGV_FT-IR_Aktionen."NOS setzen") -> ("NoOfScan"=w697:u32)  [unwired: 10 in, 7 out]
                  n328 = call "TOOLweb SET ftirScans.vi"("ftirScans"=w697) -> ()  [unwired: 2 in, 5 out]
                }
                frame #1 {
                  n329 = call "Queue LogFile.vi"() -> ("error out"=w702:errorcluster, "Queue (Ausgang)"=w701:refnum<queue>)  [unwired: 6 in]
                  n330 = call "FGV Messdaten.vi"("Aktionen"=Aktionen_FGV_Messdaten."löschen") -> ()  [unwired: 6 in, 9 out]
                  n331 = Flush Queue(queue=w701, error in (no error)=w702) -> (error out=w699:errorcluster)  [unwired: 2 out]
                  n332 = call <vilib>:"Clear Errors.vi"("error in (no error)"=w699) -> ()  [unwired: 5 in, 2 out]
                }
              }
            }
          }
          n333 = call "Zustandsfehlerinformation.vi"("Aktionen"=w682, "String"=w692) -> ("String"=w691:string)  [unwired: 9 in]
        }
      }
    }
  }
  "String für schreiben" <- w5
